vi "Home_Ref_API.vi"(0 "DVR In":refnum<data-value>, 11 "Error In":errorcluster) -> (4 "DVR Out":refnum<data-value>, 6 "VI Ref":refnum<vi>, 15 "Error Out":errorcluster)   [LabVIEW 2020, in "Test.lvclass"]
doc: "Home Reference API"
uses:
  Test.lvclass
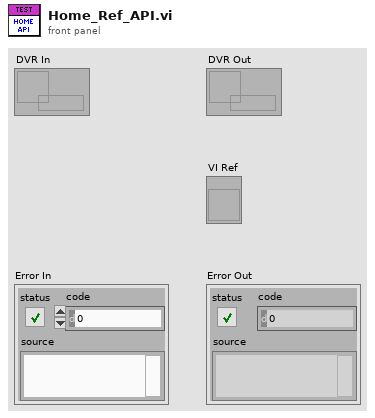
[diagram p1: front panel]
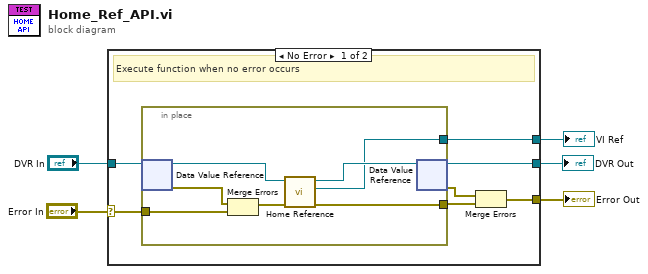
[diagram p0: block diagram]
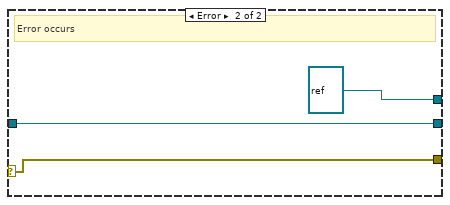
[diagram p2: hidden frame]
diagram:
  n1 = case shown="No Error" "Error In" {
    selector: "Error In" -> [w11 w22]
    tunnel: "DVR In" -> [w12 w21]
    tunnel: [w8 w22] -> w3
    tunnel: [w7 w21] -> w2
    tunnel: [w6 refnum<vi> refnum ("VI Ref")] -> w1
    frame No Error {
      # "Execute function when no error occurs"
      n2 = in-place {
        in-place-border: w11 -> [w18]
        in-place-border: [w14] -> w6
        in-place-border: [w13] -> w9
        n3 = in-place-dvr #1(w12) -> (w16:refnum<class "Test.lvclass">, w19:errorcluster)
        n4 = Merge Errors(w19, w18) -> (w17:errorcluster)
        n5 = call-dynamic "Home Reference.vi"("Error in"=w17, "Test in"=w16) -> ("Error out"=w13:errorcluster, "VI Ref"=w14:refnum<vi>, "Test out"=w15:refnum<class "Test.lvclass">)  [unwired: 7 in]
        n6 = in-place-dvr #1(w15) -> (w7:refnum<data-value>, w10:errorcluster)
      }
      n7 = Merge Errors(w10, w9) -> (w8:errorcluster)
    }
    frame Error {
      # "Error occurs"
    }
  }
  "Error Out" <- w3
  "DVR Out" <- w2
  "VI Ref" <- w1
